vi "Deviation Measurement.vi"(7 "Reference Value (0.0)":dbl min=-9.9e+37 max=9.9e+37 step=1.0 format="%.4f", 8 "error in (no error)":errorcluster, 9 "Mode (2: Off)":u32(slide)=2 max=2 step=1, 10 "Parameter (F: Secondary)":bool, 11 "VISA resource name":refnum<visa-resource-name>) -> (0 "error out":errorcluster, 3 "VISA resource name out":refnum<visa-resource-name>)   [LabVIEW 2015, in "Agilent 428X Series.lvlib"]
doc: "This function sets the deviation measurement control parameters."
uses:
  Agilent 428X Series.lvlib
panel:
  # "Primary \nSecondary"
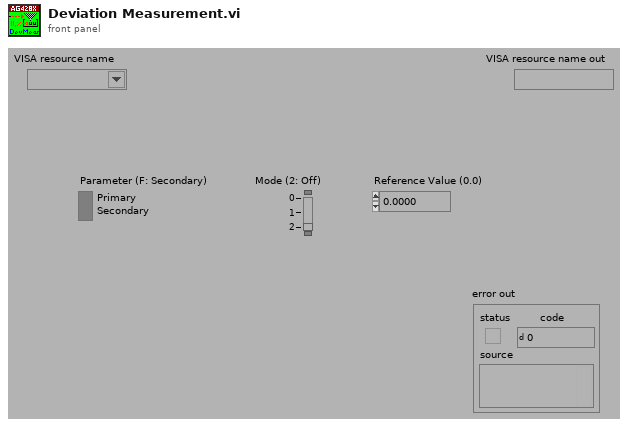
[diagram p1: front panel]
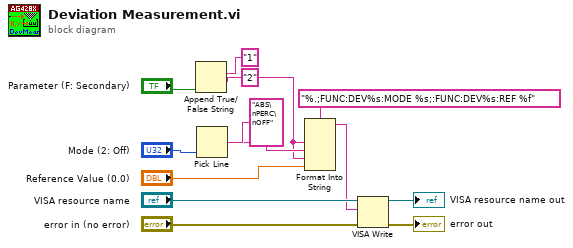
[diagram p0: block diagram]
diagram:
  n1 = Append True/False String(1:"Parameter (F: Secondary)", 2:"2" ("false string"), 3:"1" ("true string")) -> (0:w3:string)  [unwired: 1 in]
  n2 = Pick Line(multi-line string="ABS\nPERC\nOFF", line index="Mode (2: Off)") -> (output string=w4:string)  [unwired: 1 in]
  n3 = Format Into String(format string="%.;FUNC:DEV%s:MODE %s;:FUNC:DEV%s:REF %f", w3, w4, w3, "Reference Value (0.0)") -> (resulting string=w1:string)  [unwired: 2 in, 1 out]
  n4 = VISA Write(VISA resource name="VISA resource name", write buffer=w1, error in (no error)="error in (no error)") -> (VISA resource name out=→"VISA resource name out":refnum<visa-resource-name>, error out=→"error out":errorcluster)  [unwired: 1 out]
